vi "Write Index Path.vi"(8 "error in (no error)":errorcluster, 10 "Index Folder Path":path, 11 "Indexing Test Finder in":refnum<class "Indexing Test Finder.lvclass">) -> (0 "error out":errorcluster, 3 "Indexing Test Finder out":refnum<class "Indexing Test Finder.lvclass">)   [LabVIEW 2020, in "Indexing Test Finder.lvclass"]
uses:
  Indexing Test Finder.lvclass
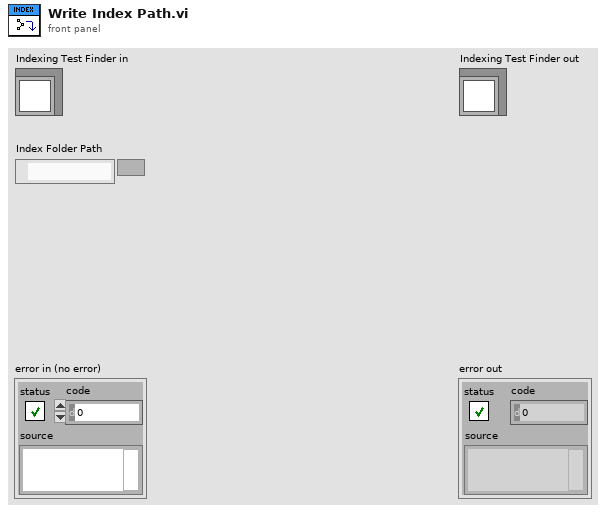
[diagram p1: front panel]
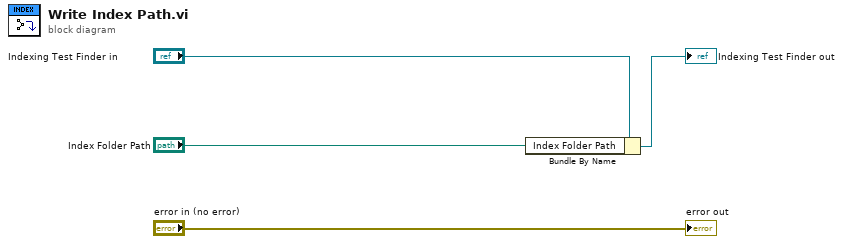
[diagram p0: block diagram]
diagram:
  n1 = Bundle By Name(cluster="Indexing Test Finder in", "Index Folder Path"="Index Folder Path") -> (→"Indexing Test Finder out":refnum<class "Indexing Test Finder.lvclass">)
  "error out" <- "error in (no error)"
